vi "Cycle History Read.vi"(0 "GEA2 Reference In":refnum<k24>, 5 "Standalone?":bool, 6 "Cycle History Buffer Selection":T1, 11 "Error In":errorcluster) -> (4 "GEA2 Reference Out":refnum<k24>, 8 "output cluster":T2, 15 "Error Out":errorcluster)   [LabVIEW 2016, in "2015 VA Washer.lvlib"]
uses:
  Projects/2015 VA Washer.lvlib
  C:/Automation/DLLs/PC Dot Net/GeaCommunication.dll
  type defs/Cycle_Diag_Teststand.ctl
  type defs/Cycle History Buffer Selector.ctl
  Common/LabVIEW GEA2 Toolkit/LabVIEW_GEA2_Toolkit.lvlibp/type defs/Source_Destination.ctl
  Common/LabVIEW GEA2 Toolkit/LabVIEW_GEA2_Toolkit.lvlibp/type defs/ERD Read Data In.ctl
  Common/LabVIEW GEA2 Toolkit/LabVIEW_GEA2_Toolkit.lvlibp/type defs/Data Type.ctl
  Common/LabVIEW GEA2 Toolkit/LabVIEW_GEA2_Toolkit.lvlibp
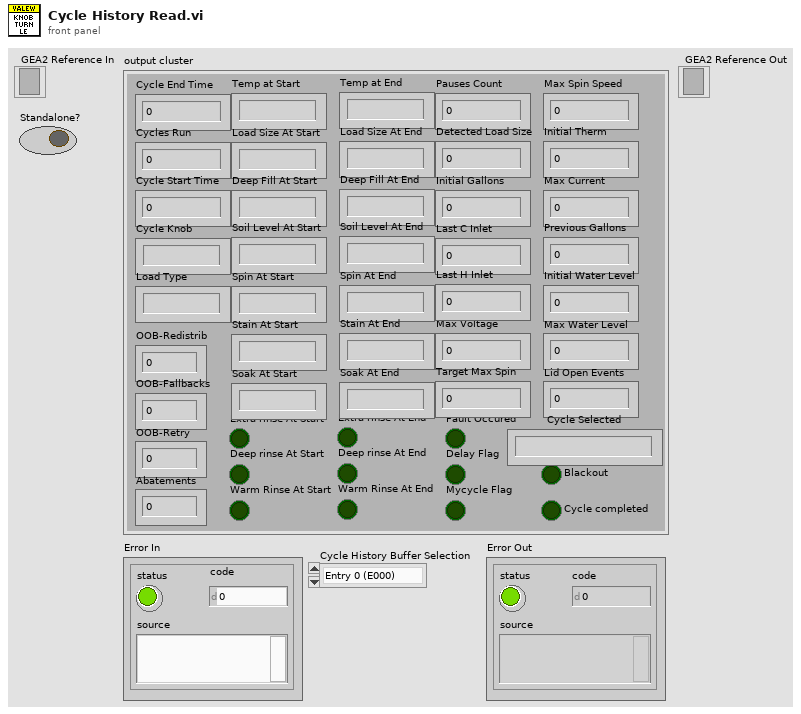
[diagram p1: front panel]
types:
  T1 = typedef "2015 VA Washer.lvlib/Cycle History Buffer Selector.ctl" = enum16{"Entry 0 (E000)", "Entry 1 (E001)", "Entry 2 (E002)", "Entry 3 (E003)", "Entry 4 (E004)", "Entry 5 (E005)", "Entry 6 (E006)", "Entry 7 (E007)", "Entry 8 (E008)", "Entry 9 (E009)"}
  T2 = typedef "2015 VA Washer.lvlib/Cycle_Diag_Teststand.ctl" = cluster{"Cycle End Time":u32, "Cycles Run":u32, "Cycle Start Time":u32, "Cycle Knob":string, "Load Type":string, "OOB-Redistrib":u8, "OOB-Fallbacks":u8, "OOB-Retry":u8, "Temp at Start":string, "Load Size At Start":string, "Deep Fill At Start":string, "Soil Level At Start":string, "Spin At Start":string, "Extra rinse At Start":bool, "Deep rinse At Start":bool, "Stain At Start":string, "Soak At Start":string, "Warm Rinse At Start":bool, "Temp at End":string, "Load Size At End":string, "Deep Fill At End":string, "Soil Level At End":string, "Spin At End":string, "Extra rinse At End":bool, "Deep rinse At End":bool, "Stain At End":string, "Soak At End":string, "Warm Rinse At End":bool, "Pauses Count":u8, "Fault Occured":bool, "Delay Flag":bool, "Mycycle Flag":bool, "Blackout":bool, "Cycle completed":bool, "Detected Load Size":dbl, "Initial Gallons":dbl, "Last C Inlet ":dbl, "Max Voltage":dbl, "Target Max Spin":u16, "Max Spin Speed":u16, "Initial Therm":dbl, "Max Current":dbl, "Previous Gallons":dbl, "Initial Water Level":dbl, "Max Water Level":dbl, "Abatements ":u8, "Lid Open Events":u8, "Cycle Selected":string, "Last H Inlet ":dbl}
  T3 = typedef "LabVIEW_GEA2_Toolkit.lvlibp/Source_Destination.ctl" = cluster{"Source":u8, "Destination":u8}
  T4 = typedef "LabVIEW_GEA2_Toolkit.lvlibp/ERD Read Data In.ctl" = cluster{"ERD Number":u16, "Data Type":T5}
  T5 = typedef "LabVIEW_GEA2_Toolkit.lvlibp/Data Type.ctl" = enum16{"string", "boolean", "uint8_t", "uint16_t", "uint32_t", "uint64_t", "int8_t", "int16_t", "int32_t", "int64_t"}
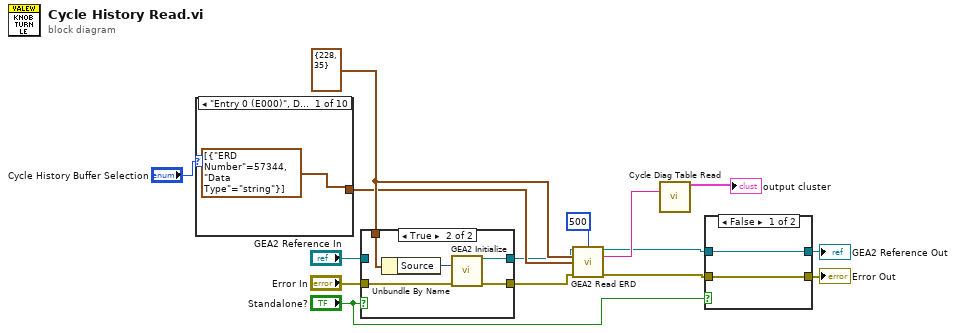
[diagram p0: block diagram]
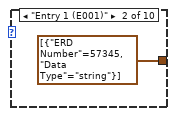
[diagram p2: hidden frame]
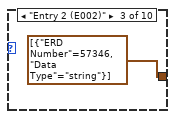
[diagram p3: hidden frame]
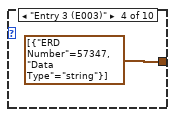
[diagram p4: hidden frame]
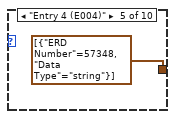
[diagram p5: hidden frame]
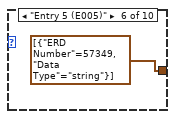
[diagram p6: hidden frame]
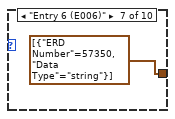
[diagram p7: hidden frame]
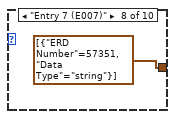
[diagram p8: hidden frame]
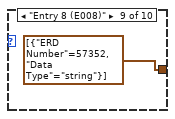
[diagram p9: hidden frame]
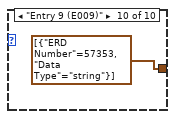
[diagram p10: hidden frame]
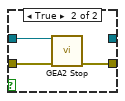
[diagram p11: hidden frame]
diagram:
  w9 = T3 {"Source"=228, "Destination"=35} ("GEA Inputs")
  n1 = case shown="\"Entry 0 (E000)\", Default" "Cycle History Buffer Selection" {
    tunnel: [T4[] [{"ERD Number"=57344, "Data Type"=enum."string"}] ("Read ERD List") T4[] [{"ERD Number"=57345, "Data Type"=enum."string"}] ("Read ERD List") T4[] [{"ERD Number"=57346, "Data Type"=enum."string"}] ("Read ERD List") T4[] [{"ERD Number"=57347, "Data Type"=enum."string"}] ("Read ERD List") T4[] [{"ERD Number"=57348, "Data Type"=enum."string"}] ("Read ERD List") T4[] [{"ERD Number"=57349, "Data Type"=enum."string"}] ("Read ERD List") T4[] [{"ERD Number"=57350, "Data Type"=enum."string"}] ("Read ERD List") T4[] [{"ERD Number"=57351, "Data Type"=enum."string"}] ("Read ERD List") T4[] [{"ERD Number"=57352, "Data Type"=enum."string"}] ("Read ERD List") T4[] [{"ERD Number"=57353, "Data Type"=enum."string"}] ("Read ERD List")] -> w7
    frame "Entry 0 (E000)", Default {
    }
    frame "Entry 1 (E001)" {
    }
    frame "Entry 2 (E002)" {
    }
    frame "Entry 3 (E003)" {
    }
    frame "Entry 4 (E004)" {
    }
    frame "Entry 5 (E005)" {
    }
    frame "Entry 6 (E006)" {
    }
    frame "Entry 7 (E007)" {
    }
    frame "Entry 8 (E008)" {
    }
    frame "Entry 9 (E009)" {
    }
  }
  n2 = case shown="True" "Standalone?" {
    tunnel: "Error In" -> [w26 w32]
    tunnel: [w26 w31] -> w10
    tunnel: "GEA2 Reference In" -> [w27 _]
    tunnel: [w27 w30] -> w6
    tunnel: w9 -> [_ w28]
    frame False {
    }
    frame True {
      n3 = Unbundle By Name(w28) -> ("Source"=w29:u8)
      n4 = call "GEA2 Initialize.vi"("Source Address"=w29, "error in"=w32) -> ("GEA2 Reference Out"=w30:refnum<k24>, "error out"=w31:errorcluster)  [unwired: 11 in, 1 out]
    }
  }
  n5 = call "GEA2 Read ERD.vi"("GEA2 Reference In"=w6, "Read Timeout (ms)"=u32 500, "GEA Inputs"=w9, "Read ERD List"=w7, "Error In"=w10) -> ("GEA2 Reference Out"=w4:refnum<k24>, "Raw Data Out"=w5:string, "Error Out"=w3:errorcluster)  [unwired: 7 in, 1 out]
  n6 = call "Cycle Diag Table Read.vi"("Raw Data In"=w5) -> ("output cluster"=→"output cluster":T2)  [unwired: 14 in]
  n7 = case shown="False" "Standalone?" {
    tunnel: [w33 w37] -> w13
    tunnel: w4 -> [w34 w36]
    tunnel: [w34 _] -> w12
    tunnel: w3 -> [w33 w35]
    frame False {
    }
    frame True {
      n8 = call "GEA2 Stop.vi"("GEA2 Reference In"=w36, "Error In"=w35) -> ("Error Out"=w37:errorcluster)  [unwired: 13 in]
    }
  }
  "Error Out" <- w13
  "GEA2 Reference Out" <- w12
